vi "Reinitial Parameter After Test.vi"(8 "error in (no error)":errorcluster, 11 "main ref":T1) -> (0 "error out":errorcluster)   [LabVIEW 2025]
uses:
  v06/controls/LAB-IQ UI Data.ctl
  Traction Loop/Traction Receipe Enum.ctl
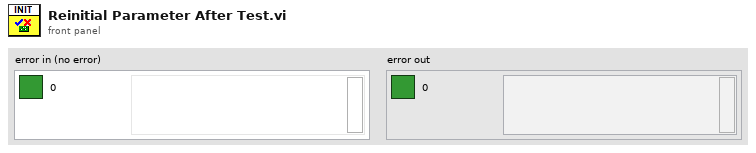
[diagram p1: front panel]
types:
  T1 = typedef "LAB-IQ UI Data.ctl" = cluster{"Main Home Screen":cluster{"GUI":refnum<vi>, "Platform Settings":refnum<vi>, "Configure":refnum<vi>, "Home":refnum<vi>, "EXIT":refnum<vi>, "service 2":refnum<vi>, "MainPage":refnum<vi>, "Analysis":refnum<vi>}, "Platform Settings":cluster{"mm/s  Surge":refnum<vi>, "Drive Error":refnum<vi>, "Disable Axis Jog Soft Limits":refnum<vi>, "mm/s  Sway":refnum<vi>, "Sway and Surge COM Status":refnum<vi>, "Heave COM Status":refnum<vi>, "Enable Platform":refnum<vi>, "Surge Forward Main":refnum<vi>, "Sway Right Main":refnum<vi>, "Sway Left Main":refnum<vi>, "Heave Down Main":refnum<vi>, "Heave Up main":refnum<vi>, "mm/s Heave":refnum<vi>, "mm/sec":refnum<vi>, "mm":refnum<vi>, "Surge Backward Main":refnum<vi>}, "Analysis Screen":cluster{"Analysis Home":refnum<vi>, "Surface Analysis":refnum<vi>, "Imaging":refnum<vi>, "Image Analysis":refnum<vi>, "Post Analysis":refnum<vi>}, "Config Screen":cluster{"Select Load Head":refnum<vi>, "Notes :":refnum<vi>, "FILE":refnum<vi>, "Sample ID :":refnum<vi>, "Operator ID :":refnum<vi>, "Operator Name :":refnum<vi>, "Auto":refnum<vi>}, "Motion Module":cluster{"zNL":refnum<vi>, "NL disp":refnum<vi>, "Rotary Tab":refnum<vi>, "Motion Direction:  3":refnum<vi>, "E.Velocity 2":refnum<vi>, "e.v/ssr 2":refnum<vi>, "Enter Fixed E.Velocity 2":refnum<vi>, "Enter Final SRR 2":refnum<vi>, "Enter initial SRR 2":refnum<vi>, "Enter Fixed SRR 2":refnum<vi>, "Enter the Final E.Velocity (m/s) 2":refnum<vi>, "Enter initial E.Velocity (m/s) 2":refnum<vi>, "Final Speed (RPM) 3":refnum<vi>, "Initial Speed (RPM) 2":refnum<vi>, "Enter the Final Velocity (m/s) 3":refnum<vi>, "Enter initial Velocity (m/s)  3":refnum<vi>, "Ramp Up 2":refnum<vi>, "TEST SELECTION":refnum<vi>, "SPEED SELECTION : ":refnum<vi>, "Angular Oscillation Set":refnum<vi>, "Traction":refnum<vi>, "Step Speed":refnum<vi>, "StepTable For Load-Speed":refnum<vi>, "StepTable For Speed":refnum<vi>, "Surge Forward MM":refnum<vi>, "Surge Backward MM":refnum<vi>, "M3 Image":refnum<vi>, "String 39":refnum<vi>, "Sway Left MM":refnum<vi>, "Sway Right MM":refnum<vi>, "Disable Axis Jog Soft Limits":refnum<vi>, "mm":refnum<vi>, "Heave Down MM":refnum<vi>, "Heave Up MM":refnum<vi>, "Wear Track Diameter (mm)":refnum<vi>, "Set WTD":refnum<vi>, "HomeScratch":refnum<vi>, "HomeRot":refnum<vi>, "PlaceModule":refnum<vi>, "Enter the Angle (Deg)":refnum<vi>, "Enter the Frequency (Hz)":refnum<vi>, "Motion Mode:":refnum<vi>, "LR Sway":refnum<vi>, "Rot Hor":refnum<vi>, "Scratch":refnum<vi>, "LR Cam":refnum<vi>, "MMBack":refnum<vi>, "MMNext":refnum<vi>, "Rot Ver":refnum<vi>, "Rotary Module Selection":refnum<vi>, "calculate rotary":refnum<vi>, "SPEED SELECTION : rotary":refnum<vi>, "Import 2":refnum<vi>, "Save 2":refnum<vi>, "File Path :  2":refnum<vi>, "String 45":refnum<vi>, "StepTable For Speed 3":refnum<vi>, "Enter the Speed(mm/sec)":refnum<vi>, "Enter the Speed(RPM)":refnum<vi>, "Enter Scratch Speed (mm/s):":refnum<vi>, "SwaySpeed Set":refnum<vi>, "Scartch Offset":refnum<vi>, "Motion type:":refnum<vi>, "HomeScratch 2":refnum<vi>, "Enter Scratch length (mm):":refnum<vi>, "Wear Track Diameter":refnum<vi>, "Rotary Speed Exced":refnum<vi>, "Scratch Mode":refnum<vi>, "No of Scratch":refnum<vi>}, "Environmental control":cluster{"Humidity  Status  3":refnum<vi>, "Low Temp  Status  2":refnum<vi>, "TK4 status 2":refnum<vi>, "Stage Temperature":refnum<vi>, "Sample Temperature":refnum<vi>, "Humidity (Amb)":refnum<vi>, "Clear List":refnum<vi>, "Add to list":refnum<vi>, "Wear":refnum<vi>, "Vibration":refnum<vi>, "Humidity (Chamber)":refnum<vi>, "Temperature (Chamber)":refnum<vi>, "ECR ":refnum<vi>, "Temperature (Amb)":refnum<vi>, "Microphone":refnum<vi>, "Acoustic Emission 3":refnum<vi>, "SNext":refnum<vi>, "APBack":refnum<vi>, "Enter the Temperature (°C):":refnum<vi>, "Enter the Stage \nTemperature (°C):":refnum<vi>, "Enter the Humidity (%Rh):":refnum<vi>, "Low Temp":refnum<vi>, "High Temp":refnum<vi>, "Humidity":refnum<vi>, "Sensors Picked":refnum<vi>}, "About Screen":cluster{"Password":refnum<vi>, "Home Service":refnum<vi>, "Advanced Setting":refnum<vi>, "About Tab":refnum<vi>, "ECR Port:":refnum<vi>, "Ramp Port:":refnum<vi>, "Installation/Replacement completed":refnum<vi>, "Loahead":refnum<vi>, "Heave and Surge COM Port:":refnum<vi>, "Sway COM Port:":refnum<vi>, "Temp Modbus:":refnum<vi>, "Humidity Port:":refnum<vi>, "Edit Gain Constants":refnum<vi>, "Save Gain Constants":refnum<vi>}, "Main Screen":cluster{"Main Screen Tab":refnum<vi>, "Angle and Frequency":refnum<vi>, "Stroke (mm)":refnum<vi>, "Angle (Deg)":refnum<vi>, "Main Speed Tab":refnum<vi>, "MTM MOTOR DISPLAY":refnum<vi>, "Disc Speed (m/sec)":refnum<vi>, "Ball Speed (m/sec)":refnum<vi>, "Disc Speed (RPM)":refnum<vi>, "Ball Speed (RPM)":refnum<vi>, "SPEED TAB":refnum<vi>, "Speed (m/sec)":refnum<vi>, "Set Speed (m/sec)":refnum<vi>, "Speed (RPM)":refnum<vi>, "Set Speed":refnum<vi>, "Time Tab":refnum<vi>, "Time ( HH:MM:SS ) 2":refnum<vi>, "Test Duration":refnum<vi>, "Test Duration 4":refnum<vi>, "TEST CYCLE":refnum<vi>, "TOTAL CYCLES":refnum<vi>, "Set Load (N)":refnum<vi>, "Temp Tabs":refnum<vi>, "Heater":refnum<vi>, "TK4 status":refnum<vi>, "ChamberTemp":refnum<vi>, "SetTmp":refnum<vi>, "Controller  Status":refnum<vi>, "ChamberTemp 2":refnum<vi>, "SetTmp 2":refnum<vi>, "Controller  Status 2":refnum<vi>, "ChamberTemp 3":refnum<vi>, "SetTmp 3":refnum<vi>, "Cooling":refnum<vi>, "Load Communication":refnum<vi>, "Ambient \nTemperature":refnum<vi>, "HumCOMStatus":refnum<vi>, "Ambient\n Humidity":refnum<vi>, "Freq (Hz)":refnum<vi>, "Load En":refnum<vi>, "NLt":refnum<vi>, "zNL 2":refnum<vi>, "Humidity On":refnum<vi>, "humidity disp":refnum<vi>, "Set Humidity":refnum<vi>, "NL disp 2":refnum<vi>, "Humidity On 2":refnum<vi>, "humidity disp 2":refnum<vi>, "Set Humidity 2":refnum<vi>, "NL disp 3":refnum<vi>, "AppLoadSeq scratch":refnum<vi>, "Stop Scratch":refnum<vi>, "ClrLog":refnum<vi>, "Trip Log":refnum<vi>, "STOP":refnum<vi>, "Start Test":refnum<vi>, "Test status":refnum<vi>, "AR Led":refnum<vi>, "Data":refnum<vi>, "Health":refnum<vi>, "Sway COM Status":refnum<vi>, "Heave COM Status":refnum<vi>, "Grp Tab":refnum<vi>, "Sub Graph":refnum<vi>, "SD (mm)":refnum<vi>, "Siliding distance Reset Graph":refnum<vi>, "SDGp":refnum<vi>, "Humidity Reset Graph":refnum<vi>, "HumrGp":refnum<vi>, "Acoustic Emission (mV)":refnum<vi>, "Aqucostic Reset Graph":refnum<vi>, "gACQUOS":refnum<vi>, "ECR RESET":refnum<vi>, "ECR":refnum<vi>, "Temperature Reset":refnum<vi>, "Acoustic Emission (mV) 2":refnum<vi>, "Aqucostic Reset Graph 2":refnum<vi>, "gACQUOS 2":refnum<vi>, "ECR RESET 2":refnum<vi>, "ECR 2":refnum<vi>, "Temperature Reset 2":refnum<vi>, "Temperature (deg c)":refnum<vi>, "Speed Reset Graph":refnum<vi>, "Speed Tab":refnum<vi>, "MTM DISC  SPEED":refnum<vi>, "MTM BALL SPEED":refnum<vi>, "speed mm/sec":refnum<vi>, "Hymidity":refnum<vi>, "Humidity Disable trip":refnum<vi>, "CoF Trip  2":refnum<vi>, "Depth Trip":refnum<vi>, "Weart Deapth":refnum<vi>, "Depth Reset Graph":refnum<vi>, "Weart":refnum<vi>, "Depthz":refnum<vi>, "Depth (µm)":refnum<vi>, "WearGp":refnum<vi>, "NL Trip 2":refnum<vi>, "Load pid":refnum<vi>, "Load Disable Trip":refnum<vi>, "Load Reset Graph":refnum<vi>, "NL Display 4":refnum<vi>, "Main Chart 3":refnum<vi>, "BACK":refnum<vi>, "Depth Trip 2":refnum<vi>, "COF TRIP ":refnum<vi>, "Friction Force (N)":refnum<vi>, "FF Reset Graph":refnum<vi>, "FF Disable Trip":refnum<vi>, "FF TRIP":refnum<vi>, "COF Disable Trip":refnum<vi>, "COF Reset Graph":refnum<vi>, "Start Test Temp":refnum<vi>, "zFF":refnum<vi>, "Friction Force (N) Graph":refnum<vi>, "Coefficient of Friction":refnum<vi>, "Scratch Start Test":refnum<vi>, "FF Tab":refnum<vi>, "Cyclic Friction Force (N)":refnum<vi>, "CZ FF":refnum<vi>, "Cyclic Friction Force (N) Graph":refnum<vi>, "Cyclic Coefficient of Friction":refnum<vi>, "Cyclic FF TRIP":refnum<vi>, "Cyclic FF Disable Trip":refnum<vi>, "cyclic COF Disable Trip":refnum<vi>, "cyclic COF TRIP":refnum<vi>, "cyclic COF Reset Graph":refnum<vi>, "Cyclic FF Reset Graph":refnum<vi>, "Test Trip":refnum<vi>, "Multi Scratch Pass":refnum<vi>, "Scratch Start Recording":refnum<vi>, "Coefficient of Friction 2":refnum<vi>, "Acoustic Emission":refnum<vi>, "Friction Force (N) 2":refnum<vi>, "Depth (Microns)":refnum<vi>, "Normal Load ( N )":refnum<vi>}, "Loading":cluster{"Indentation":refnum<vi>, "Reference Sample":refnum<vi>, "Load Cell Communication Slide":refnum<vi>, "com 3":refnum<vi>, "com":refnum<vi>, "DecaForce COM Status":refnum<vi>, "Update":refnum<vi>, "Clear 3":refnum<vi>, "seq":refnum<vi>, "Stribeck table":refnum<vi>, "Stribeck Table  For loading":refnum<vi>, "Loading Mode":refnum<vi>, "Enter the Final Load (N)":refnum<vi>, "Enter the CoF Trip":refnum<vi>, "Enter the Friction Force Trip":refnum<vi>, "Enter the Normal load Trip":refnum<vi>, "Enter the Load  (N)":refnum<vi>, "KiloForce":refnum<vi>, "DecaForce ":refnum<vi>, "MicroForce":refnum<vi>, "LHBack":refnum<vi>, "LHNext":refnum<vi>, "Enter the Loading Rate (N/min)":refnum<vi>, "Message":refnum<vi>, "Warning 2":refnum<vi>, "SSP 0.75":refnum<vi>, "SSP 0.5":refnum<vi>, "SSP 0.3":refnum<vi>, "Warning":refnum<vi>, "gui GIF":refnum<vi>, "Communication is established":refnum<vi>, "AppLoad 4":refnum<vi>, "Multipoint":refnum<vi>, "Load Selection":refnum<vi>}, "PID":cluster{"Ramp":refnum<vi>, "Vertical load (N)":refnum<vi>, "apply load":refnum<vi>, "apply load 2":refnum<vi>, "Enter ByPass Load":refnum<vi>, "Bypass Load":refnum<vi>, "gFF Rot":refnum<vi>}, "Config Parameters":cluster{"Tab Control 3":refnum<vi>, "Tab Control 19":refnum<vi>, "SAMPLES":refnum<vi>, "Re-initilaize":refnum<vi>, "Filter ON/OFF":refnum<vi>, "TracHomeSurgeOffsetCounts 10MM":refnum<vi>, "TracHomeSwayOffsetCounts 10MM":refnum<vi>, "Acoustic Emission:":refnum<vi>, "Apply Filter (FF)":refnum<vi>, "Filter% 2":refnum<vi>, "Apply Filter (Load)":refnum<vi>, "Filter% ":refnum<vi>, "Sway distance (mm)":refnum<vi>, "Surge distance (mm)":refnum<vi>, "DataSavingLoopDelay(ms)":refnum<vi>, "SAVE 2":refnum<vi>, "Enter Distance":refnum<vi>, "Sway Counts:":refnum<vi>, "Distance (mm): 3":refnum<vi>, "Surge Counts:":refnum<vi>, "Distance (mm): 2":refnum<vi>, "Distance (mm):":refnum<vi>, "Heave Counts:":refnum<vi>, "LRMHomeSurgeOffsetCounts":refnum<vi>, "LRMHomeSwayOffsetCounts":refnum<vi>, "TracHomeSurgeOffsetCounts 20MM":refnum<vi>, "TracHomeSwayOffsetCounts 20MM":refnum<vi>, "RotHomeSwayOffsetCounts":refnum<vi>, "RotHomeSurgeOffsetCounts":refnum<vi>, "Heave distance":refnum<vi>, "Zmm":refnum<vi>, "Heave Pulses/mm":refnum<vi>, "Surge Pulses/mm":refnum<vi>, "Sway Pulses/mm":refnum<vi>, "Heave Pitch":refnum<vi>, "Surge Pitch":refnum<vi>, "Sway Pitch":refnum<vi>, "Heave PPR":refnum<vi>, "Surge PPR":refnum<vi>, "Sway PPR":refnum<vi>, "Tab Control 5":refnum<vi>, "Tab Control 14":refnum<vi>, "Tab Control 26":refnum<vi>, "AE":refnum<vi>, "Heave Loop Delay":refnum<vi>, "Heave PID Speed":refnum<vi>, "Surge Jog Speed":refnum<vi>, "Heave Jog Speed":refnum<vi>, "Sway Loop Delay":refnum<vi>, "Sway PID Speed":refnum<vi>, "Sway Jog Speed":refnum<vi>, "DEPTH TRIP VALUE":refnum<vi>, "LOAD TRIP VALUE":refnum<vi>, "DEPTH TRIP   ENABLE":refnum<vi>, "LOAD TRIP  ENABLE":refnum<vi>, "CYCLIC FF TRIP VALUE":refnum<vi>, "FF TRIP VALUE":refnum<vi>, "CYCLIC CoF TRIP VALUE":refnum<vi>, "COF TRIP VALUE":refnum<vi>, "CYCLIC COF TRIP  ENABLE":refnum<vi>, "CYCLIC FF TRIP  ENABLE":refnum<vi>, "FF TRIP  ENABLE":refnum<vi>, "COF TRIP  ENABLE":refnum<vi>, "JOG TRIP LOAD VALUE (N)":refnum<vi>, "Rotary Vertical":refnum<vi>, "Traction":refnum<vi>, "Scratch":refnum<vi>, "LRM CAM":refnum<vi>, "Sway LRM":refnum<vi>, "Rotary Horizontal":refnum<vi>, "SURGE SPEED":refnum<vi>, "SURGE BACKWARD COUNT":refnum<vi>, "SURGE FORWARD COUNT":refnum<vi>, "Start Button":refnum<vi>}, "Loading Com Port":cluster{"ClearAll":refnum<vi>, "Mz(Nm)":refnum<vi>, "My(Nm)":refnum<vi>, "Mx(Nm)":refnum<vi>, "Save Dwell":refnum<vi>, "Acq Delay (ms)":refnum<vi>, "Burst Delay (ms)":refnum<vi>, "model":refnum<vi>, "SN":refnum<vi>, "FFx(N)":refnum<vi>, "Sensor IP":refnum<vi>, "Port":refnum<vi>, "FFy(N)":refnum<vi>, "Load(N)":refnum<vi>, "delete Handle":refnum<vi>, "Create Handle":refnum<vi>, "ft_data":refnum<vi>, "ft_range":refnum<vi>, "ft_data 2":refnum<vi>, "stop 6":refnum<vi>, "running_flag":refnum<vi>, "ft_udp_handle":refnum<vi>, "get-data-return":refnum<vi>, "get-range-return":refnum<vi>, "zero-return":refnum<vi>, "filter-return":refnum<vi>, "initial-return":refnum<vi>, "deleteHandle-result":refnum<vi>, "Load Cell Temp":refnum<vi>, "Load Cell":refnum<vi>, "ZeroAll":refnum<vi>, "FORCE (N)":refnum<vi>, "TORQUE (N-m)":refnum<vi>, "Load Cell Link":refnum<vi>}, "Heave AND Surge":cluster{"SURGE POSE":refnum<vi>, "error out Read":refnum<vi>, "HEAVE POSE":refnum<vi>, "State":refnum<vi>, "Homed":refnum<vi>, "Sequence ID":refnum<vi>, "error out Write":refnum<vi>, "faultCode":refnum<vi>, "Ack ID":refnum<vi>, "SPEED":refnum<vi>, "Distance":refnum<vi>, "Mode Command":refnum<vi>, "Heave and Surge Read":refnum<vi>, "Read Heave Temp":refnum<vi>, "Spare 15":refnum<vi>, "Spare 14":refnum<vi>, "Spare 13":refnum<vi>, "Spare 12":refnum<vi>, "Spare 11":refnum<vi>, "Spare 10":refnum<vi>, "Spare 9":refnum<vi>, "Spare 8":refnum<vi>, "Spare 7":refnum<vi>, "Spare 4":refnum<vi>, "Spare 3":refnum<vi>, "Spare 2":refnum<vi>, "Humidity":refnum<vi>, "Temp":refnum<vi>, "Node Id":refnum<vi>, "Spare 1":refnum<vi>, "SPARE 4":refnum<vi>, "SPARE 3":refnum<vi>, "SPARE 2":refnum<vi>, "SPARE 1":refnum<vi>, "fwMajor":refnum<vi>, "fwMinor":refnum<vi>, "Manual Write":refnum<vi>, "Heave and Surge Write":refnum<vi>, "SPARE 5":refnum<vi>, "Reserved ":refnum<vi>, "SPARE 8":refnum<vi>, "SPARE 6":refnum<vi>, "SPARE 7":refnum<vi>, "SPARE 17":refnum<vi>, "SPARE 16":refnum<vi>, "SPARE 15":refnum<vi>, "SPARE 14":refnum<vi>, "SPARE 13":refnum<vi>, "SPARE 12":refnum<vi>, "SPARE 11":refnum<vi>, "SPARE 10":refnum<vi>, "SPARE 9":refnum<vi>, "System UPTIME":refnum<vi>, "Missed Packets":refnum<vi>, "faultCode Surge Right":refnum<vi>, "faultCode Surge Left":refnum<vi>, "faultCode Heave":refnum<vi>, "UPLINK HEAVE":refnum<vi>, "DOWNLINK HEAVE":refnum<vi>}, "New PID LOGIC":cluster{"Fine Tune Zone":refnum<vi>, "PID SDelay":refnum<vi>, "Max_pos_limit":refnum<vi>, "Min_pos_limit":refnum<vi>, "i_limit":refnum<vi>, "pct_scale":refnum<vi>, "Deadband":refnum<vi>, "Kd":refnum<vi>, "Ki":refnum<vi>, "Kp":refnum<vi>, "Current Position":refnum<vi>, "Set Load":refnum<vi>, "Current Load":refnum<vi>, "Pulse delta":refnum<vi>, "Init Step":refnum<vi>, "Max Step Linit":refnum<vi>, "min_deadband_floor":refnum<vi>, "dynamic_spindle_noise_scalar":refnum<vi>, "min_finetune_floor":refnum<vi>, "filter_alpha":refnum<vi>, "PID":refnum<vi>}, "SWAY ":cluster{"fwMajor":refnum<vi>, "Homed":refnum<vi>, "Rotary POSE":refnum<vi>, "State":refnum<vi>, "SWAY POSE":refnum<vi>, "Ack ID":refnum<vi>, "faultCode":refnum<vi>, "Node Id":refnum<vi>, "fwMinor":refnum<vi>, "Spare 6":refnum<vi>, "Spare 5":refnum<vi>, "Spare 4":refnum<vi>, "Spare 3":refnum<vi>, "Spare 2":refnum<vi>, "Spare 1":refnum<vi>, "Spare 7":refnum<vi>, "SPARE  5":refnum<vi>, "error out Write  SWAY ":refnum<vi>, "error out Read SWAY ":refnum<vi>, "Manual Write SWAY ":refnum<vi>, "SWAY WRITE":refnum<vi>, "SPARE  4":refnum<vi>, "SPARE  3":refnum<vi>, "SPARE 2":refnum<vi>, "SPARE 1":refnum<vi>, "Spare 15":refnum<vi>, "Spare 14":refnum<vi>, "Spare 13":refnum<vi>, "Spare 12":refnum<vi>, "Spare 11":refnum<vi>, "Spare 9":refnum<vi>, "Spare 8":refnum<vi>, "SPEED":refnum<vi>, "Distance":refnum<vi>, "Mode Command":refnum<vi>, "Sequence ID":refnum<vi>, "SWAY READ":refnum<vi>, "Spare 10":refnum<vi>, "Read SWAY Temp":refnum<vi>, "faultCode Sway ":refnum<vi>, "Missed Packets":refnum<vi>, "System UPTIME sway":refnum<vi>, "SPARE 6":refnum<vi>, "SPARE 7":refnum<vi>, "SPARE 9":refnum<vi>, "SPARE 11":refnum<vi>, "SPARE 10":refnum<vi>, "SPARE 8":refnum<vi>, "SPARE 13":refnum<vi>, "SPARE 12":refnum<vi>, "SPARE 17":refnum<vi>, "SPARE 16":refnum<vi>, "SPARE 15":refnum<vi>, "SPARE 14":refnum<vi>, "Reserved":refnum<vi>, "faultCode Rotary":refnum<vi>, "UPLINK SWAY":refnum<vi>, "DOWNLINK SWAY":refnum<vi>}, "Analysis Screen":cluster{"Analysis Home":refnum<vi>, "Refresh 2":refnum<vi>, "MEAN 4":refnum<vi>, "SD 4":refnum<vi>, "VARIANCE 4":refnum<vi>, "MEAN  3":refnum<vi>, "SD  3":refnum<vi>, "VARIANCE  3":refnum<vi>, "MEAN 2":refnum<vi>, "SD  2":refnum<vi>, "VARIANCE 2":refnum<vi>, "MEAN":refnum<vi>, "SD":refnum<vi>, "VARIANCE":refnum<vi>, "File 4 Discription":refnum<vi>, "OPEN 4":refnum<vi>, "File Name 4":refnum<vi>, "OPEN 3":refnum<vi>, "File 3 Discription":refnum<vi>, "File Name 3":refnum<vi>, "Y-AXIS":refnum<vi>, "X-AXIS":refnum<vi>, "XY Graph":refnum<vi>, "File Name 2":refnum<vi>, "File Name 1":refnum<vi>, "OPEN 2":refnum<vi>, "OPEN 1":refnum<vi>, "File 1 Discription ":refnum<vi>, "File 2 Discription":refnum<vi>, "Export":refnum<vi>, "File Format":refnum<vi>}, "Traction":cluster{"faultCode Traction 2":refnum<vi>, "faultCode Traction 1":refnum<vi>, "Missed Packets":refnum<vi>, "System UPTIME Traction":refnum<vi>, "SPARE 17":refnum<vi>, "SPARE 16":refnum<vi>, "SPARE 15":refnum<vi>, "SPARE 14":refnum<vi>, "SPARE 13":refnum<vi>, "SPARE 12":refnum<vi>, "SPARE 11":refnum<vi>, "SPARE 10":refnum<vi>, "SPARE 9":refnum<vi>, "SPARE 8":refnum<vi>, "SPARE 7":refnum<vi>, "SPARE 6":refnum<vi>, "Reserved":refnum<vi>, "SPARE  5":refnum<vi>, "Manual Write TRACTION":refnum<vi>, "TRACTION WRITE":refnum<vi>, "SPARE  4":refnum<vi>, "SPARE  3":refnum<vi>, "SPARE 2":refnum<vi>, "SPARE 1":refnum<vi>, "Spare 7":refnum<vi>, "Spare 6":refnum<vi>, "Spare 5":refnum<vi>, "Spare 4":refnum<vi>, "Spare 2":refnum<vi>, "Spare 1":refnum<vi>, "Node Id":refnum<vi>, "Read TRACTION Temp":refnum<vi>, "fwMinor":refnum<vi>, "fwMajor":refnum<vi>, "faultCode":refnum<vi>, "TRACTION POSE":refnum<vi>, "TRACTION POSE 2":refnum<vi>, "Homed":refnum<vi>, "State":refnum<vi>, "Ack ID":refnum<vi>, "SPEED":refnum<vi>, "Distance":refnum<vi>, "Mode Command":refnum<vi>, "Sequence ID":refnum<vi>, "error out Read TRACTION":refnum<vi>, "error out Write  TRACTION":refnum<vi>, "TRACTION READ":refnum<vi>, "Spare 3":refnum<vi>, "Downlink traction":refnum<vi>, "Uplink Traction":refnum<vi>}, "Traction reciepe":cluster{"SRR Sweep Range (%) Stribeck":refnum<vi>, "Traction Receipe":refnum<vi>, "Total Execution Time":refnum<vi>, "Total Steps":refnum<vi>, "Duration / Step (s)  Stribeck":refnum<vi>, "STRIBECK Fixed SRR List (%)":refnum<vi>, "Duration / Step (s) Traction":refnum<vi>, "SRR Sweep Range (%) traction":refnum<vi>, "Rolling Speed (mm/s)":refnum<vi>, "Temperature Stages (°C)":refnum<vi>, "Ball Load (N)":refnum<vi>, "Lubricant Name":refnum<vi>, "Profile File Name":refnum<vi>, "SET entrainment Velocity":refnum<vi>, "Test Array Size":refnum<vi>, "SRR INDEX [ STRIBECK]":refnum<vi>, "Stribeck Size":refnum<vi>, "SET SRR":refnum<vi>, "ELAPSED TIMER ":refnum<vi>, "BALL SET RPM":refnum<vi>, "DISC SET RPM":refnum<vi>, "SET LOAD":refnum<vi>, "TEMPERATURE READ":refnum<vi>, "SET TEMPERATURE":refnum<vi>, "Traction Size":refnum<vi>, "DISC SPEED (rpm)":refnum<vi>, "BALL SPEED (rpm)":refnum<vi>, "BALL WEAR TRACK":refnum<vi>, "DISC WEARTRACK":refnum<vi>, "SRR INDEX [ TRACTION]":refnum<vi>, "Start Index Type":refnum<vi>, "Enum - Menu":refnum<vi>, "Ball (mm/sec)":refnum<vi>, "Disc (mm/sec)":refnum<vi>, "Traction Receipe Update Details":refnum<vi>}, "Traction Control":cluster{"HomeTraction":refnum<vi>, "Demo Mode Display":refnum<vi>, "Traction Message":refnum<vi>, "Traction Step Update Details":refnum<vi>, "Main Tab sequence for selection":refnum<vi>, "Ramp Tab":refnum<vi>, "e.v/ssr":refnum<vi>, "Enter Fixed E.Velocity":refnum<vi>, "Enter Final SRR":refnum<vi>, "Enter initial SRR":refnum<vi>, "Enter Fixed SRR":refnum<vi>, "Enter the Final E.Velocity (m/s)":refnum<vi>, "Enter initial E.Velocity (m/s)":refnum<vi>, "Ball WTD":refnum<vi>, "E.Velocity":refnum<vi>, "Enter the Final Velocity (m/s)":refnum<vi>, "Enter initial Velocity (m/s)":refnum<vi>, "Ramp Up   Disc":refnum<vi>, "Initial DiscSpeed (RPM)":refnum<vi>, "Final Speed (RPM) Ball":refnum<vi>, "Final Speed (RPM)":refnum<vi>, "Initial Speed (RPM) Ball":refnum<vi>, "Enter the Final Velocity (m/s) Ball":refnum<vi>, "Enter initial Velocity (m/s) Ball":refnum<vi>, "Ramp Up":refnum<vi>, "ExceedBallSpeed step":refnum<vi>, "ExceedDiscSpeed":refnum<vi>, "BallSpeed Exceed Indication":refnum<vi>, "Apply":refnum<vi>, "SPEED SELECTION : MTM":refnum<vi>, "SPEED SELECTION : MTM 2":refnum<vi>, "TEST SELECTION (MTM)":refnum<vi>, "MTM Test Selection":refnum<vi>, "File Path Tab":refnum<vi>, "File Path String":refnum<vi>, "Save":refnum<vi>, "Save  2":refnum<vi>, "Import ":refnum<vi>, "File Path :":refnum<vi>, "Step Sequence Indication Tab":refnum<vi>, "Step Sequence Indication":refnum<vi>, "Calculate Step":refnum<vi>, "StepTable":refnum<vi>, "ExceedDiscSpeed  Cinstant Speed":refnum<vi>, "ExceedBallSpeed Constant":refnum<vi>, "TEST SELECTION (MTM) 2":refnum<vi>, "SPEED SELECTION : MTM 3":refnum<vi>, "MTM Test Selection 2":refnum<vi>, "Enter the Speed (m/sec): ":refnum<vi>, "Enter the Speed (m/sec):  2":refnum<vi>, "Enter the Speed (RPM):":refnum<vi>, "Lower Spped ":refnum<vi>, "Upper":refnum<vi>, "Enter the Speed (RPM):Ball":refnum<vi>, "Disc Motion Direction: ":refnum<vi>, "Ball Motion Direction :":refnum<vi>, "Motion Mode: ":refnum<vi>, "Wear Track Diameter (mm) ":refnum<vi>, "Disc Speed Indicator":refnum<vi>, "ExceedBallSpeed":refnum<vi>}, "Acquostic":cluster{"Last Config Rejected ":refnum<vi>, "rx command count":refnum<vi>, "Current Filter Id":refnum<vi>, "Isolated Gain":refnum<vi>, "DAQ Status":refnum<vi>, "error out":refnum<vi>, "error in (no error)":refnum<vi>, "Uplink Packet":refnum<vi>, "data out":refnum<vi>, "Downlink Packet":refnum<vi>, "Gains":refnum<vi>, "Manual Write Acquostic":refnum<vi>, "Acoustic Graphs":refnum<vi>}, "ABOUT":cluster{"version":refnum<vi>, "Operating System":refnum<vi>, "Version":refnum<vi>, "Workorder":refnum<vi>, "Runtime":refnum<vi>, "Instrument Serial":refnum<vi>, "Firmware Version":refnum<vi>, "Info":refnum<vi>}, "Temperature Port":cluster{"Temperature":refnum<vi>, "error out Temperature":refnum<vi>, "READ TEMPERATURE":refnum<vi>}}
  T2 = enum8{"Enabled", "Disabled", "Disabled and Grayed Out"}
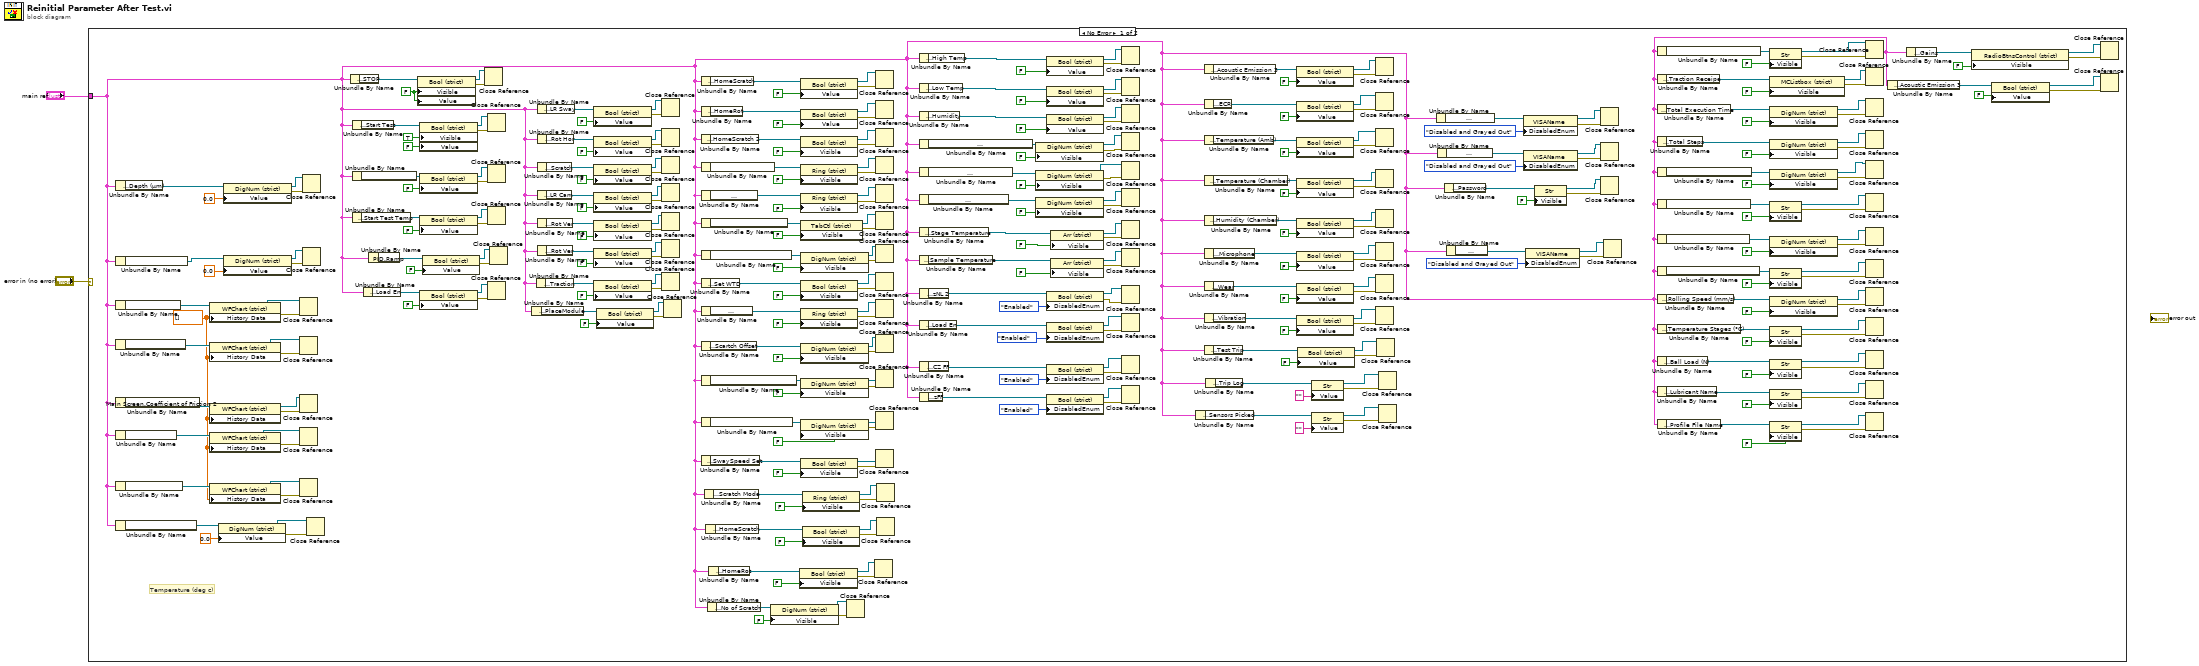
[diagram p0: block diagram]
diagram:
  n1 = case shown="No Error" "error in (no error)" {
    tunnel: "main ref" -> [w5 _]
    frame No Error {
      w4 = dbl[] [] ("History Data")
      w301 = FALSE ("Visible")
      # "Temperature (deg c)"
      n2 = Unbundle By Name(w5) -> ("Main Screen.Depth (µm)"=w323:refnum<vi>)
      n3 = Unbundle By Name(w5) -> ("Main Screen.Time ( HH:MM:SS ) 2"=w319:refnum<vi>)
      n4 = Unbundle By Name(w5) -> ("Main Screen.Normal Load ( N )"=w23:refnum<vi>)
      n5 = Unbundle By Name(w5) -> ("Main Screen.Friction Force (N) 2"=w20:refnum<vi>)
      n6 = Unbundle By Name(w5) -> ("Main Screen.Coefficient of Friction 2"=w17:refnum<vi>)
      n7 = Unbundle By Name(w5) -> ("Main Screen.Depth (Microns)"=w14:refnum<vi>)
      n8 = Unbundle By Name(w5) -> ("Main Screen.Acoustic Emission"=w11:refnum<vi>)
      n9 = Unbundle By Name(w5) -> ("Main Screen.Acoustic Emission (mV)"=w6:refnum<vi>)
      n10 = property on="Property Node" class="WFChart (strict)"(reference=w23, "History Data"=w4) -> (reference out=w21:refnum<vi>, error out=w22:errorcluster)  [unwired: 1 in]
      n11 = property on="Property Node" class="WFChart (strict)"(reference=w20, "History Data"=w4) -> (reference out=w18:refnum<vi>, error out=w19:errorcluster)  [unwired: 1 in]
      n12 = property on="Property Node" class="WFChart (strict)"(reference=w17, "History Data"=w4) -> (reference out=w15:refnum<vi>, error out=w16:errorcluster)  [unwired: 1 in]
      n13 = property on="Property Node" class="WFChart (strict)"(reference=w14, "History Data"=w4) -> (reference out=w12:refnum<vi>, error out=w13:errorcluster)  [unwired: 1 in]
      n14 = property on="Property Node" class="WFChart (strict)"(reference=w11, "History Data"=w4) -> (reference out=w9:refnum<vi>, error out=w10:errorcluster)  [unwired: 1 in]
      n15 = property on="Property Node" class="DigNum (strict)"(reference=w6, "Value"=0.0) -> (reference out=w8:refnum<vi>, error out=w7:errorcluster)  [unwired: 1 in]
      n16 = property class="DigNum (strict)"(reference=w323, "Value"=0.0) -> (reference out=w324:refnum<vi>, error out=w322:errorcluster)  [unwired: 1 in]
      n17 = property class="DigNum (strict)"(reference=w319, "Value"=0.0) -> (reference out=w317:refnum<vi>, error out=w320:errorcluster)  [unwired: 1 in]
      n18 = Close Reference(reference=w21, error in (no error)=w22) -> ()  [unwired: 1 out]
      n19 = Close Reference(reference=w18, error in (no error)=w19) -> ()  [unwired: 1 out]
      n20 = Close Reference(reference=w15, error in (no error)=w16) -> ()  [unwired: 1 out]
      n21 = Close Reference(reference=w12, error in (no error)=w13) -> ()  [unwired: 1 out]
      n22 = Close Reference(reference=w9, error in (no error)=w10) -> ()  [unwired: 1 out]
      n23 = Close Reference(reference=w324, error in (no error)=w322) -> ()  [unwired: 1 out]
      n24 = Close Reference(reference=w317, error in (no error)=w320) -> ()  [unwired: 1 out]
      n25 = Close Reference(reference=w8, error in (no error)=w7) -> ()  [unwired: 1 out]
      n26 = Unbundle By Name(w5) -> ("Main Screen.STOP"=w307:refnum<vi>)
      n27 = Unbundle By Name(w5) -> ("Main Screen.Start Test"=w305:refnum<vi>)
      n28 = Unbundle By Name(w5) -> ("Main Screen.Scratch Start Test"=w313:refnum<vi>)
      n29 = Unbundle By Name(w5) -> ("Main Screen.Start Test Temp"=w314:refnum<vi>)
      n30 = Unbundle By Name(w5) -> ("Main Screen.Load En"=w293:refnum<vi>)
      n31 = Unbundle By Name(w5) -> ("PID.Ramp"=w298:refnum<vi>)
      n32 = property class="Bool (strict)"(reference=w307, "Visible"=w301, "Value"=w301) -> (reference out=w302:refnum<vi>, error out=w308:errorcluster)  [unwired: 1 in]
      n33 = property class="Bool (strict)"(reference=w305, "Visible"=TRUE, "Value"=FALSE) -> (reference out=w303:refnum<vi>, error out=w304:errorcluster)  [unwired: 1 in]
      n34 = property class="Bool (strict)"(reference=w313, "Value"=FALSE) -> (reference out=w311:refnum<vi>, error out=w312:errorcluster)  [unwired: 1 in]
      n35 = property class="Bool (strict)"(reference=w314, "Value"=FALSE) -> (reference out=w316:refnum<vi>, error out=w315:errorcluster)  [unwired: 1 in]
      n36 = property class="Bool (strict)"(reference=w293, "Value"=FALSE) -> (reference out=w295:refnum<vi>, error out=w294:errorcluster)  [unwired: 1 in]
      n37 = property class="Bool (strict)"(reference=w298, "Value"=FALSE) -> (reference out=w296:refnum<vi>, error out=w297:errorcluster)  [unwired: 1 in]
      n38 = Close Reference(reference=w302, error in (no error)=w308) -> ()  [unwired: 1 out]
      n39 = Close Reference(reference=w303, error in (no error)=w304) -> ()  [unwired: 1 out]
      n40 = Close Reference(reference=w311, error in (no error)=w312) -> ()  [unwired: 1 out]
      n41 = Close Reference(reference=w316, error in (no error)=w315) -> ()  [unwired: 1 out]
      n42 = Close Reference(reference=w295, error in (no error)=w294) -> ()  [unwired: 1 out]
      n43 = Close Reference(reference=w296, error in (no error)=w297) -> ()  [unwired: 1 out]
      n44 = Unbundle By Name(w5) -> ("Motion Module.PlaceModule"=w262:refnum<vi>)
      n45 = Unbundle By Name(w5) -> ("Motion Module.Traction"=w266:refnum<vi>)
      n46 = Unbundle By Name(w5) -> ("Motion Module.LR Sway"=w289:refnum<vi>)
      n47 = Unbundle By Name(w5) -> ("Motion Module.Rot Hor"=w286:refnum<vi>)
      n48 = Unbundle By Name(w5) -> ("Motion Module.Scratch"=w282:refnum<vi>)
      n49 = Unbundle By Name(w5) -> ("Motion Module.LR Cam"=w277:refnum<vi>)
      n50 = Unbundle By Name(w5) -> ("Motion Module.Rot Ver"=w274:refnum<vi>)
      n51 = Unbundle By Name(w5) -> ("Motion Module.Rot Ver"=w270:refnum<vi>)
      n52 = property class="Bool (strict)"(reference=w289, "Value"=FALSE) -> (reference out=w291:refnum<vi>, error out=w290:errorcluster)  [unwired: 1 in]
      n53 = property class="Bool (strict)"(reference=w286, "Value"=FALSE) -> (reference out=w284:refnum<vi>, error out=w285:errorcluster)  [unwired: 1 in]
      n54 = property class="Bool (strict)"(reference=w282, "Value"=FALSE) -> (reference out=w280:refnum<vi>, error out=w283:errorcluster)  [unwired: 1 in]
      n55 = property class="Bool (strict)"(reference=w277, "Value"=FALSE) -> (reference out=w279:refnum<vi>, error out=w276:errorcluster)  [unwired: 1 in]
      n56 = property class="Bool (strict)"(reference=w274, "Value"=FALSE) -> (reference out=w272:refnum<vi>, error out=w275:errorcluster)  [unwired: 1 in]
      n57 = property class="Bool (strict)"(reference=w270, "Value"=FALSE) -> (reference out=w268:refnum<vi>, error out=w269:errorcluster)  [unwired: 1 in]
      n58 = property class="Bool (strict)"(reference=w266, "Value"=FALSE) -> (reference out=w264:refnum<vi>, error out=w265:errorcluster)  [unwired: 1 in]
      n59 = property class="Bool (strict)"(reference=w262, "Value"=FALSE) -> (reference out=w260:refnum<vi>, error out=w261:errorcluster)  [unwired: 1 in]
      n60 = Close Reference(reference=w291, error in (no error)=w290) -> ()  [unwired: 1 out]
      n61 = Close Reference(reference=w284, error in (no error)=w285) -> ()  [unwired: 1 out]
      n62 = Close Reference(reference=w280, error in (no error)=w283) -> ()  [unwired: 1 out]
      n63 = Close Reference(reference=w279, error in (no error)=w276) -> ()  [unwired: 1 out]
      n64 = Close Reference(reference=w272, error in (no error)=w275) -> ()  [unwired: 1 out]
      n65 = Close Reference(reference=w268, error in (no error)=w269) -> ()  [unwired: 1 out]
      n66 = Close Reference(reference=w264, error in (no error)=w265) -> ()  [unwired: 1 out]
      n67 = Close Reference(reference=w260, error in (no error)=w261) -> ()  [unwired: 1 out]
      n68 = Unbundle By Name(w5) -> ("Motion Module.HomeScratch"=w230:refnum<vi>)
      n69 = Unbundle By Name(w5) -> ("Motion Module.HomeRot"=w233:refnum<vi>)
      n70 = Unbundle By Name(w5) -> ("Motion Module.HomeScratch 2"=w237:refnum<vi>)
      n71 = Unbundle By Name(w5) -> ("Motion Module.Motion Direction:  3"=w242:refnum<vi>)
      n72 = Unbundle By Name(w5) -> ("Motion Module.Motion Mode:"=w245:refnum<vi>)
      n73 = Unbundle By Name(w5) -> ("Motion Module.Rotary Module Selection"=w249:refnum<vi>)
      n74 = Unbundle By Name(w5) -> ("Motion Module.Wear Track Diameter (mm)"=w253:refnum<vi>)
      n75 = Unbundle By Name(w5) -> ("Motion Module.Set WTD"=w257:refnum<vi>)
      n76 = Unbundle By Name(w5) -> ("Motion Module.Motion type:"=w226:refnum<vi>)
      n77 = Unbundle By Name(w5) -> ("Motion Module.Scartch Offset"=w223:refnum<vi>)
      n78 = Unbundle By Name(w5) -> ("Motion Module.Enter Scratch Speed (mm/s):"=w218:refnum<vi>)
      n79 = Unbundle By Name(w5) -> ("Motion Module.Enter Scratch length (mm):"=w214:refnum<vi>)
      n80 = Unbundle By Name(w5) -> ("Motion Module.SwaySpeed Set"=w210:refnum<vi>)
      n81 = Unbundle By Name(w5) -> ("Motion Module.Scratch Mode"=w159:refnum<vi>)
      n82 = Unbundle By Name(w5) -> ("Motion Module.HomeScratch"=w154:refnum<vi>)
      n83 = Unbundle By Name(w5) -> ("Motion Module.No of Scratch"=w86:refnum<vi>)
      n84 = Unbundle By Name(w5) -> ("Motion Module.HomeRot"=w151:refnum<vi>)
      n85 = property class="DigNum (strict)"(reference=w86, "Visible"=FALSE) -> (reference out=w87:refnum<vi>, error out=w85:errorcluster)  [unwired: 1 in]
      n86 = property class="Bool (strict)"(reference=w151, "Visible"=FALSE ("Value")) -> (reference out=w149:refnum<vi>, error out=w152:errorcluster)  [unwired: 1 in]
      n87 = property class="Bool (strict)"(reference=w230, "Value"=FALSE) -> (reference out=w228:refnum<vi>, error out=w229:errorcluster)  [unwired: 1 in]
      n88 = property class="Bool (strict)"(reference=w233, "Value"=FALSE) -> (reference out=w235:refnum<vi>, error out=w234:errorcluster)  [unwired: 1 in]
      n89 = property class="Bool (strict)"(reference=w237, "Visible"=FALSE ("Value")) -> (reference out=w239:refnum<vi>, error out=w236:errorcluster)  [unwired: 1 in]
      n90 = property class="Ring (strict)"(reference=w242, "Visible"=FALSE ("Value")) -> (reference out=w240:refnum<vi>, error out=w243:errorcluster)  [unwired: 1 in]
      n91 = property class="Ring (strict)"(reference=w245, "Visible"=FALSE ("Value")) -> (reference out=w247:refnum<vi>, error out=w244:errorcluster)  [unwired: 1 in]
      n92 = property class="TabCtl (strict)"(reference=w249, "Visible"=FALSE ("Value")) -> (reference out=w251:refnum<vi>, error out=w250:errorcluster)  [unwired: 1 in]
      n93 = property class="DigNum (strict)"(reference=w253, "Visible"=FALSE ("Value")) -> (reference out=w255:refnum<vi>, error out=w254:errorcluster)  [unwired: 1 in]
      n94 = property class="Bool (strict)"(reference=w257, "Visible"=FALSE ("Value")) -> (reference out=w259:refnum<vi>, error out=w258:errorcluster)  [unwired: 1 in]
      n95 = property class="Ring (strict)"(reference=w226, "Visible"=FALSE ("Value")) -> (reference out=w221:refnum<vi>, error out=w225:errorcluster)  [unwired: 1 in]
      n96 = property class="DigNum (strict)"(reference=w223, "Visible"=FALSE ("Value")) -> (reference out=w220:refnum<vi>, error out=w222:errorcluster)  [unwired: 1 in]
      n97 = property class="DigNum (strict)"(reference=w218, "Visible"=FALSE ("Value")) -> (reference out=w216:refnum<vi>, error out=w217:errorcluster)  [unwired: 1 in]
      n98 = property class="DigNum (strict)"(reference=w214, "Visible"=FALSE ("Value")) -> (reference out=w212:refnum<vi>, error out=w213:errorcluster)  [unwired: 1 in]
      n99 = property class="Bool (strict)"(reference=w210, "Visible"=FALSE ("Value")) -> (reference out=w208:refnum<vi>, error out=w209:errorcluster)  [unwired: 1 in]
      n100 = property class="Ring (strict)"(reference=w159, "Visible"=FALSE ("Value")) -> (reference out=w157:refnum<vi>, error out=w160:errorcluster)  [unwired: 1 in]
      n101 = property class="Bool (strict)"(reference=w154, "Visible"=FALSE ("Value")) -> (reference out=w156:refnum<vi>, error out=w153:errorcluster)  [unwired: 1 in]
      n102 = Close Reference(reference=w87, error in (no error)=w85) -> ()  [unwired: 1 out]
      n103 = Close Reference(reference=w149, error in (no error)=w152) -> ()  [unwired: 1 out]
      n104 = Close Reference(reference=w228, error in (no error)=w229) -> ()  [unwired: 1 out]
      n105 = Close Reference(reference=w235, error in (no error)=w234) -> ()  [unwired: 1 out]
      n106 = Close Reference(reference=w239, error in (no error)=w236) -> ()  [unwired: 1 out]
      n107 = Close Reference(reference=w240, error in (no error)=w243) -> ()  [unwired: 1 out]
      n108 = Close Reference(reference=w247, error in (no error)=w244) -> ()  [unwired: 1 out]
      n109 = Close Reference(reference=w251, error in (no error)=w250) -> ()  [unwired: 1 out]
      n110 = Close Reference(reference=w255, error in (no error)=w254) -> ()  [unwired: 1 out]
      n111 = Close Reference(reference=w259, error in (no error)=w258) -> ()  [unwired: 1 out]
      n112 = Close Reference(reference=w221, error in (no error)=w225) -> ()  [unwired: 1 out]
      n113 = Close Reference(reference=w220, error in (no error)=w222) -> ()  [unwired: 1 out]
      n114 = Close Reference(reference=w216, error in (no error)=w217) -> ()  [unwired: 1 out]
      n115 = Close Reference(reference=w212, error in (no error)=w213) -> ()  [unwired: 1 out]
      n116 = Close Reference(reference=w208, error in (no error)=w209) -> ()  [unwired: 1 out]
      n117 = Close Reference(reference=w157, error in (no error)=w160) -> ()  [unwired: 1 out]
      n118 = Close Reference(reference=w156, error in (no error)=w153) -> ()  [unwired: 1 out]
      n119 = Unbundle By Name(w5) -> ("Environmental control.High Temp"=w178:refnum<vi>)
      n120 = Unbundle By Name(w5) -> ("Environmental control.Low Temp"=w181:refnum<vi>)
      n121 = Unbundle By Name(w5) -> ("Environmental control.Humidity"=w185:refnum<vi>)
      n122 = Unbundle By Name(w5) -> ("Environmental control.Enter the Stage \nTemperature (°C):"=w190:refnum<vi>)
      n123 = Unbundle By Name(w5) -> ("Environmental control.Enter the Temperature (°C):"=w193:refnum<vi>)
      n124 = Unbundle By Name(w5) -> ("Environmental control.Enter the Humidity (%Rh):"=w197:refnum<vi>)
      n125 = Unbundle By Name(w5) -> ("Environmental control.Stage Temperature"=w201:refnum<vi>)
      n126 = Unbundle By Name(w5) -> ("Environmental control.Sample Temperature"=w205:refnum<vi>)
      n127 = Unbundle By Name(w5) -> ("Main Screen.zNL 2"=w176:refnum<vi>)
      n128 = Unbundle By Name(w5) -> ("Main Screen.Load En"=w172:refnum<vi>)
      n129 = Unbundle By Name(w5) -> ("Main Screen.CZ FF"=w166:refnum<vi>)
      n130 = Unbundle By Name(w5) -> ("Main Screen.zFF"=w163:refnum<vi>)
      n131 = property class="DigNum (strict)"(reference=w190, "Visible"=FALSE ("Value")) -> (reference out=w188:refnum<vi>, error out=w191:errorcluster)  [unwired: 1 in]
      n132 = property class="DigNum (strict)"(reference=w193, "Visible"=FALSE ("Value")) -> (reference out=w195:refnum<vi>, error out=w192:errorcluster)  [unwired: 1 in]
      n133 = property class="DigNum (strict)"(reference=w197, "Visible"=FALSE ("Value")) -> (reference out=w199:refnum<vi>, error out=w198:errorcluster)  [unwired: 1 in]
      n134 = property class="Bool (strict)"(reference=w178, "Value"=FALSE) -> (reference out=w148:refnum<vi>, error out=w177:errorcluster)  [unwired: 1 in]
      n135 = property class="Bool (strict)"(reference=w181, "Value"=FALSE) -> (reference out=w183:refnum<vi>, error out=w182:errorcluster)  [unwired: 1 in]
      n136 = property class="Bool (strict)"(reference=w185, "Value"=FALSE) -> (reference out=w187:refnum<vi>, error out=w184:errorcluster)  [unwired: 1 in]
      n137 = property class="Bool (strict)"(reference=w176, "DisabledEnum"=T2."Enabled" ("Disabled")) -> (reference out=w174:refnum<vi>, error out=w175:errorcluster)  [unwired: 1 in]
      n138 = property class="Bool (strict)"(reference=w172, "DisabledEnum"=T2."Enabled" ("Disabled")) -> (reference out=w170:refnum<vi>, error out=w171:errorcluster)  [unwired: 1 in]
      n139 = property class="Bool (strict)"(reference=w166, "DisabledEnum"=T2."Enabled" ("Disabled")) -> (reference out=w165:refnum<vi>, error out=w167:errorcluster)  [unwired: 1 in]
      n140 = property class="Bool (strict)"(reference=w163, "DisabledEnum"=T2."Enabled" ("Disabled")) -> (reference out=w164:refnum<vi>, error out=w162:errorcluster)  [unwired: 1 in]
      n141 = property class="Arr (strict)"(reference=w201, "Visible"=FALSE ("Value")) -> (reference out=w203:refnum<vi>, error out=w202:errorcluster)  [unwired: 1 in]
      n142 = property class="Arr (strict)"(reference=w205, "Visible"=FALSE ("Value")) -> (reference out=w207:refnum<vi>, error out=w206:errorcluster)  [unwired: 1 in]
      n143 = Close Reference(reference=w148, error in (no error)=w177) -> ()  [unwired: 1 out]
      n144 = Close Reference(reference=w183, error in (no error)=w182) -> ()  [unwired: 1 out]
      n145 = Close Reference(reference=w187, error in (no error)=w184) -> ()  [unwired: 1 out]
      n146 = Close Reference(reference=w188, error in (no error)=w191) -> ()  [unwired: 1 out]
      n147 = Close Reference(reference=w195, error in (no error)=w192) -> ()  [unwired: 1 out]
      n148 = Close Reference(reference=w199, error in (no error)=w198) -> ()  [unwired: 1 out]
      n149 = Close Reference(reference=w203, error in (no error)=w202) -> ()  [unwired: 1 out]
      n150 = Close Reference(reference=w207, error in (no error)=w206) -> ()  [unwired: 1 out]
      n151 = Close Reference(reference=w174, error in (no error)=w175) -> ()  [unwired: 1 out]
      n152 = Close Reference(reference=w170, error in (no error)=w171) -> ()  [unwired: 1 out]
      n153 = Close Reference(reference=w165, error in (no error)=w167) -> ()  [unwired: 1 out]
      n154 = Close Reference(reference=w164, error in (no error)=w162) -> ()  [unwired: 1 out]
      n155 = Unbundle By Name(w5) -> ("Environmental control.Sensors Picked"=w105:refnum<vi>)
      n156 = Unbundle By Name(w5) -> ("Environmental control.Acoustic Emission 3"=w146:refnum<vi>)
      n157 = Unbundle By Name(w5) -> ("Environmental control.ECR"=w142:refnum<vi>)
      n158 = Unbundle By Name(w5) -> ("Environmental control.Temperature (Amb)"=w140:refnum<vi>)
      n159 = Unbundle By Name(w5) -> ("Environmental control.Temperature (Chamber)"=w137:refnum<vi>)
      n160 = Unbundle By Name(w5) -> ("Environmental control.Humidity (Chamber)"=w134:refnum<vi>)
      n161 = Unbundle By Name(w5) -> ("Environmental control.Microphone"=w131:refnum<vi>)
      n162 = Unbundle By Name(w5) -> ("Environmental control.Wear"=w128:refnum<vi>)
      n163 = Unbundle By Name(w5) -> ("Environmental control.Vibration"=w125:refnum<vi>)
      n164 = Unbundle By Name(w5) -> ("Main Screen.Test Trip"=w114:refnum<vi>)
      n165 = Unbundle By Name(w5) -> ("Main Screen.Trip Log"=w110:refnum<vi>)
      n166 = property class="Bool (strict)"(reference=w146, "Value"=FALSE) -> (reference out=w147:refnum<vi>, error out=w145:errorcluster)  [unwired: 1 in]
      n167 = property class="Bool (strict)"(reference=w142, "Value"=FALSE) -> (reference out=w144:refnum<vi>, error out=w143:errorcluster)  [unwired: 1 in]
      n168 = property class="Bool (strict)"(reference=w140, "Value"=FALSE) -> (reference out=w139:refnum<vi>, error out=w141:errorcluster)  [unwired: 1 in]
      n169 = property class="Bool (strict)"(reference=w137, "Value"=FALSE) -> (reference out=w138:refnum<vi>, error out=w136:errorcluster)  [unwired: 1 in]
      n170 = property class="Bool (strict)"(reference=w134, "Value"=FALSE) -> (reference out=w133:refnum<vi>, error out=w135:errorcluster)  [unwired: 1 in]
      n171 = property class="Bool (strict)"(reference=w131, "Value"=FALSE) -> (reference out=w132:refnum<vi>, error out=w130:errorcluster)  [unwired: 1 in]
      n172 = property class="Bool (strict)"(reference=w128, "Value"=FALSE) -> (reference out=w127:refnum<vi>, error out=w129:errorcluster)  [unwired: 1 in]
      n173 = property class="Bool (strict)"(reference=w125, "Value"=FALSE) -> (reference out=w126:refnum<vi>, error out=w124:errorcluster)  [unwired: 1 in]
      n174 = property class="Bool (strict)"(reference=w114, "Value"=FALSE) -> (reference out=w115:refnum<vi>, error out=w113:errorcluster)  [unwired: 1 in]
      n175 = property class="Str"(reference=w110, "Value"="") -> (reference out=w109:refnum<vi>, error out=w111:errorcluster)  [unwired: 1 in]
      n176 = property class="Str"(reference=w105, "Value"="") -> (reference out=w106:refnum<vi>, error out=w104:errorcluster)  [unwired: 1 in]
      n177 = Close Reference(reference=w147, error in (no error)=w145) -> ()  [unwired: 1 out]
      n178 = Close Reference(reference=w144, error in (no error)=w143) -> ()  [unwired: 1 out]
      n179 = Close Reference(reference=w139, error in (no error)=w141) -> ()  [unwired: 1 out]
      n180 = Close Reference(reference=w138, error in (no error)=w136) -> ()  [unwired: 1 out]
      n181 = Close Reference(reference=w133, error in (no error)=w135) -> ()  [unwired: 1 out]
      n182 = Close Reference(reference=w132, error in (no error)=w130) -> ()  [unwired: 1 out]
      n183 = Close Reference(reference=w127, error in (no error)=w129) -> ()  [unwired: 1 out]
      n184 = Close Reference(reference=w126, error in (no error)=w124) -> ()  [unwired: 1 out]
      n185 = Close Reference(reference=w115, error in (no error)=w113) -> ()  [unwired: 1 out]
      n186 = Close Reference(reference=w109, error in (no error)=w111) -> ()  [unwired: 1 out]
      n187 = Close Reference(reference=w106, error in (no error)=w104) -> ()  [unwired: 1 out]
      n188 = Unbundle By Name(w5) -> ("About Screen.Temp Modbus:"=w102:refnum<vi>)
      n189 = Unbundle By Name(w5) -> ("About Screen.Humidity Port:"=w101:refnum<vi>)
      n190 = Unbundle By Name(w5) -> ("About Screen.Password"=w96:refnum<vi>)
      n191 = Unbundle By Name(w5) -> ("About Screen.ECR Port:"=w91:refnum<vi>)
      n192 = property class="VISAName"(reference=w102, "DisabledEnum"=T2."Disabled and Grayed Out" ("Disabled")) -> (reference out=w92:refnum<vi>, error out=w103:errorcluster)  [unwired: 1 in]
      n193 = property class="VISAName"(reference=w101, "DisabledEnum"=T2."Disabled and Grayed Out" ("Disabled")) -> (reference out=w99:refnum<vi>, error out=w100:errorcluster)  [unwired: 1 in]
      n194 = property class="VISAName"(reference=w91, "DisabledEnum"=T2."Disabled and Grayed Out" ("Disabled")) -> (reference out=w88:refnum<vi>, error out=w90:errorcluster)  [unwired: 1 in]
      n195 = property class="Str"(reference=w96, "Visible"=FALSE) -> (reference out=w98:refnum<vi>, error out=w97:errorcluster)  [unwired: 1 in]
      n196 = Close Reference(reference=w92, error in (no error)=w103) -> ()  [unwired: 1 out]
      n197 = Close Reference(reference=w99, error in (no error)=w100) -> ()  [unwired: 1 out]
      n198 = Close Reference(reference=w98, error in (no error)=w97) -> ()  [unwired: 1 out]
      n199 = Close Reference(reference=w88, error in (no error)=w90) -> ()  [unwired: 1 out]
      n200 = Unbundle By Name(w5) -> ("Traction reciepe.SRR Sweep Range (%) Stribeck"=w66:refnum<vi>)
      n201 = Unbundle By Name(w5) -> ("Traction reciepe.Traction Receipe"=w69:refnum<vi>)
      n202 = Unbundle By Name(w5) -> ("Traction reciepe.Total Execution Time"=w72:refnum<vi>)
      n203 = Unbundle By Name(w5) -> ("Traction reciepe.Total Steps"=w64:refnum<vi>)
      n204 = Unbundle By Name(w5) -> ("Traction reciepe.Duration / Step (s)  Stribeck"=w61:refnum<vi>)
      n205 = Unbundle By Name(w5) -> ("Traction reciepe.STRIBECK Fixed SRR List (%)"=w58:refnum<vi>)
      n206 = Unbundle By Name(w5) -> ("Traction reciepe.Duration / Step (s) Traction"=w81:refnum<vi>)
      n207 = Unbundle By Name(w5) -> ("Traction reciepe.SRR Sweep Range (%) traction"=w45:refnum<vi>)
      n208 = Unbundle By Name(w5) -> ("Traction reciepe.Rolling Speed (mm/s)"=w42:refnum<vi>)
      n209 = Unbundle By Name(w5) -> ("Traction reciepe.Temperature Stages (°C)"=w39:refnum<vi>)
      n210 = Unbundle By Name(w5) -> ("Traction reciepe.Ball Load (N)"=w47:refnum<vi>)
      n211 = Unbundle By Name(w5) -> ("Traction reciepe.Lubricant Name"=w50:refnum<vi>)
      n212 = Unbundle By Name(w5) -> ("Traction reciepe.Profile File Name"=w53:refnum<vi>)
      n213 = property class="Str"(reference=w66, "Visible"=FALSE) -> (reference out=w67:refnum<vi>, error out=w65:errorcluster)  [unwired: 1 in]
      n214 = property class="MCListbox (strict)"(reference=w69, "Visible"=FALSE) -> (reference out=w68:refnum<vi>, error out=w70:errorcluster)  [unwired: 1 in]
      n215 = property class="DigNum (strict)"(reference=w72, "Visible"=FALSE) -> (reference out=w73:refnum<vi>, error out=w71:errorcluster)  [unwired: 1 in]
      n216 = property class="DigNum (strict)"(reference=w64, "Visible"=FALSE) -> (reference out=w59:refnum<vi>, error out=w63:errorcluster)  [unwired: 1 in]
      n217 = property class="DigNum (strict)"(reference=w61, "Visible"=FALSE) -> (reference out=w60:refnum<vi>, error out=w62:errorcluster)  [unwired: 1 in]
      n218 = property class="Str"(reference=w58, "Visible"=FALSE) -> (reference out=w56:refnum<vi>, error out=w57:errorcluster)  [unwired: 1 in]
      n219 = property class="DigNum (strict)"(reference=w81, "Visible"=FALSE) -> (reference out=w83:refnum<vi>, error out=w82:errorcluster)  [unwired: 1 in]
      n220 = property class="Str"(reference=w45, "Visible"=FALSE) -> (reference out=w44:refnum<vi>, error out=w46:errorcluster)  [unwired: 1 in]
      n221 = property class="DigNum (strict)"(reference=w42, "Visible"=FALSE) -> (reference out=w43:refnum<vi>, error out=w41:errorcluster)  [unwired: 1 in]
      n222 = property class="Str"(reference=w39, "Visible"=FALSE) -> (reference out=w38:refnum<vi>, error out=w40:errorcluster)  [unwired: 1 in]
      n223 = property class="Str"(reference=w47, "Visible"=FALSE) -> (reference out=w52:refnum<vi>, error out=w48:errorcluster)  [unwired: 1 in]
      n224 = property class="Str"(reference=w50, "Visible"=FALSE) -> (reference out=w51:refnum<vi>, error out=w49:errorcluster)  [unwired: 1 in]
      n225 = property class="Str"(reference=w53, "Visible"=FALSE) -> (reference out=w55:refnum<vi>, error out=w54:errorcluster)  [unwired: 1 in]
      n226 = Close Reference(reference=w67, error in (no error)=w65) -> ()  [unwired: 1 out]
      n227 = Close Reference(reference=w68, error in (no error)=w70) -> ()  [unwired: 1 out]
      n228 = Close Reference(reference=w73, error in (no error)=w71) -> ()  [unwired: 1 out]
      n229 = Close Reference(reference=w59, error in (no error)=w63) -> ()  [unwired: 1 out]
      n230 = Close Reference(reference=w60, error in (no error)=w62) -> ()  [unwired: 1 out]
      n231 = Close Reference(reference=w56, error in (no error)=w57) -> ()  [unwired: 1 out]
      n232 = Close Reference(reference=w83, error in (no error)=w82) -> ()  [unwired: 1 out]
      n233 = Close Reference(reference=w44, error in (no error)=w46) -> ()  [unwired: 1 out]
      n234 = Close Reference(reference=w43, error in (no error)=w41) -> ()  [unwired: 1 out]
      n235 = Close Reference(reference=w38, error in (no error)=w40) -> ()  [unwired: 1 out]
      n236 = Close Reference(reference=w52, error in (no error)=w48) -> ()  [unwired: 1 out]
      n237 = Close Reference(reference=w51, error in (no error)=w49) -> ()  [unwired: 1 out]
      n238 = Close Reference(reference=w55, error in (no error)=w54) -> ()  [unwired: 1 out]
      n239 = Unbundle By Name(w5) -> ("Environmental control.Acoustic Emission 3"=w29:refnum<vi>)
      n240 = Unbundle By Name(w5) -> ("Acquostic.Gains"=w28:refnum<vi>)
      n241 = property class="RadioBtnsControl (strict)"(reference=w28, "Visible"=FALSE) -> (reference out=w24:refnum<vi>, error out=w27:errorcluster)  [unwired: 1 in]
      n242 = property class="Bool (strict)"(reference=w29, "Value"=FALSE ("Visible")) -> (reference out=w31:refnum<vi>, error out=w30:errorcluster)  [unwired: 1 in]
      n243 = Close Reference(reference=w24, error in (no error)=w27) -> ()  [unwired: 1 out]
      n244 = Close Reference(reference=w31, error in (no error)=w30) -> ()  [unwired: 1 out]
    }
    frame Error {
    }
  }
